vi "Load Data.vi"(8 "error in (no error)":errorcluster) -> (0 "error out":errorcluster, 2 "Sound WAV data":waveform(dbl)[](array[waveform]), 3 "Wind Data":dbl[][](array[numeric]))   [LabVIEW 2019]
uses:
  <vilib>/Utility/file.llb/Read Delimited Spreadsheet (DBL).vi
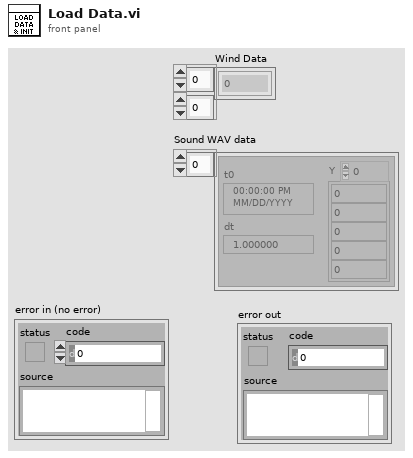
[diagram p1: front panel]
types:
  T1 = enum32{"invalid app kind", "Development System", "Run Time System", "Student Edition", "Embedded LabVIEW", "Evaluation", "Custom"}
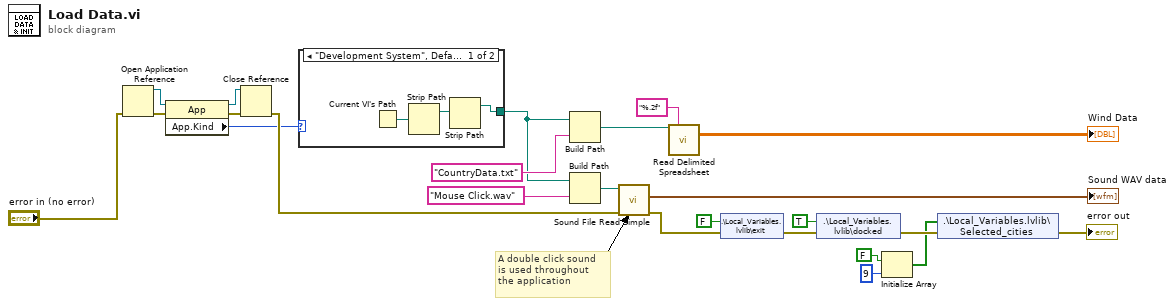
[diagram p0: block diagram]
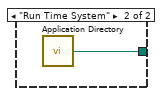
[diagram p2: hidden frame]
diagram:
  # "A double click sound\nis used throughout\nthe application"
  n1 = Open Application Reference(8:"error in (no error)") -> (0:w9:errorcluster, 3:w10:refnum<vi>)  [unwired: 3 in]
  n2 = property class="App"(reference=w10, error in=w9) -> (reference out=w8:refnum<vi>, error out=w7:errorcluster, "App.Kind"=w4:T1)
  n3 = Close Reference(reference=w8, error in (no error)=w7) -> (error out=w5:errorcluster)
  n4 = case shown="\"Development System\", Default" w4 {
    tunnel: [w25 w28] -> w1
    frame "Development System", Default {
      n5 = Current VI's Path() -> (path=w27:path)
      n6 = Strip Path(path=w27) -> (stripped path=w26:path)  [unwired: 1 out]
      n7 = Strip Path(path=w26) -> (stripped path=w25:path)  [unwired: 1 out]
    }
    frame "Run Time System" {
      n8 = call <vilib>:"Application Directory.vi"() -> ("Application Directory"=w28:path)
    }
  }
  n9 = Build Path(base path=w1, name or relative path="CountryData.txt") -> (appended path=w3:path)
  n10 = Build Path(base path=w1, name or relative path="Mouse Click.wav") -> (appended path=w2:path)
  n11 = call <vilib>:"Sound File Read Simple.vi"("error in (no error)"=w5, "path"=w2) -> ("error out"=w18:errorcluster, "data"=→"Sound WAV data":waveform(dbl)[])  [unwired: 6 in, 2 out]
  n12 = call-poly <vilib>:"Read Delimited Spreadsheet.vi"("file path (dialog if empty)"=w3, "format (%.3f)"="%.2f") -> ("all rows"=→"Wind Data":dbl[][])  [unwired: 8 in, 5 out]
  n13 = shared-variable ".\\Local_Variables.lvlib\\exit"(FALSE ("exit"), error in=w18) -> (error out=w17:errorcluster)
  n14 = shared-variable ".\\Local_Variables.lvlib\\docked"(TRUE ("docked"), error in=w17) -> (error out=w15:errorcluster)
  n15 = Initialize Array(FALSE, 9 ("dimension size")) -> (w13:bool[])
  n16 = shared-variable ".\\Local_Variables.lvlib\\Selected_cities"(w13, error in=w15) -> (error out=→"error out":errorcluster)
